vi "Set Delay Generator.vi"(9 "typ":i32, 10 "address":i16, 11 "board":i32) -> (3 "function return":u32)   [LabVIEW 2018, in "Copy of Andor SDK.lvlib"]
doc: "EXPNETTYPE unsigned int WINAPI SetDelayGenerator(int board, short address, int typ);"
uses:
  Copy of Andor SDK.lvlib
  <userlib>/Andor SDK/ATMCD32D.dll
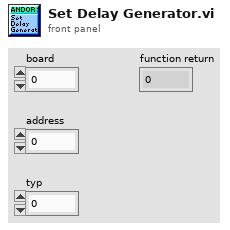
[diagram p1: front panel]
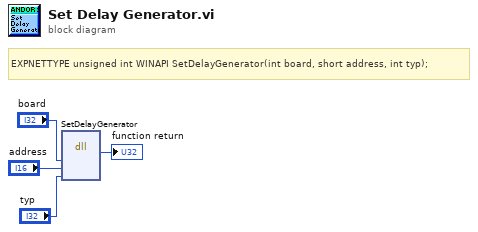
[diagram p0: block diagram]
diagram:
  # "EXPNETTYPE unsigned int WINAPI SetDelayGenerator(int board, short address, int typ);"
  n1 = dll-call lib="C:/Program Files (x86)/National Instruments/LabVIEW 2018/user.lib/Andor SDK/ATMCD32D.*" fn="SetDelayGenerator"("board"="board", "address"="address", "typ"="typ") -> (→"function return":u32)  [unwired: 6 in, 2 out]
